vi "DB Tools Free Object.vi"   [LabVIEW 2020, in "NI_Database_API.lvlib"]
doc: "Frees an object by destroying its associated reference and returns a different reference object. Wire data to the reference input to determine the polymorphic instance to use or manually select the instance."
uses:
  <vilib>/addons/database/NI_Database_API.lvlib
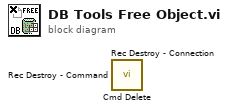
[diagram p0: block diagram]
diagram:
  n1 = call <vilib>:"Cmd Delete.vi"() -> ()  [unwired: 10 in, 2 out]
  n2 = call <vilib>:"Rec Destroy - Connection.vi"() -> ()  [unwired: 10 in, 2 out]
  n3 = call <vilib>:"Rec Destroy - Command.vi"() -> ()  [unwired: 10 in, 2 out]
